vi "DB Set Measurement.vi"(4 "KH serial number":string, 5 "measurement":string, 6 "lockin serial number":string, 7 "device":string, 8 "error in (no error)":errorcluster, 9 "Station":string, 10 "User":string) -> (0 "error out":errorcluster)   [LabVIEW 2019, in "Control Experiment.lvclass"]
uses:
  Control Experiment.lvclass
  <userlib>/LevyLab/LV-Data/LV-Data.PG/LV-Data.PGSQL.lvclass
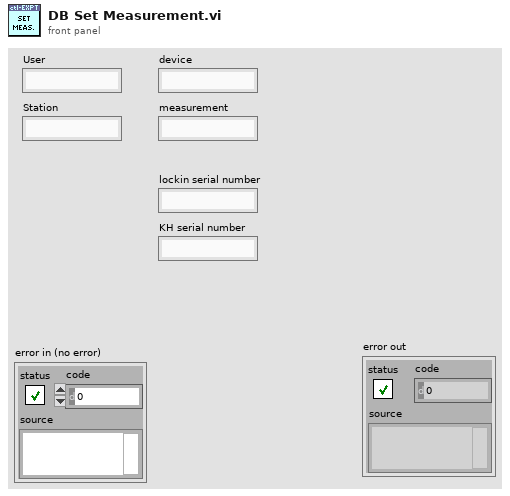
[diagram p1: front panel]
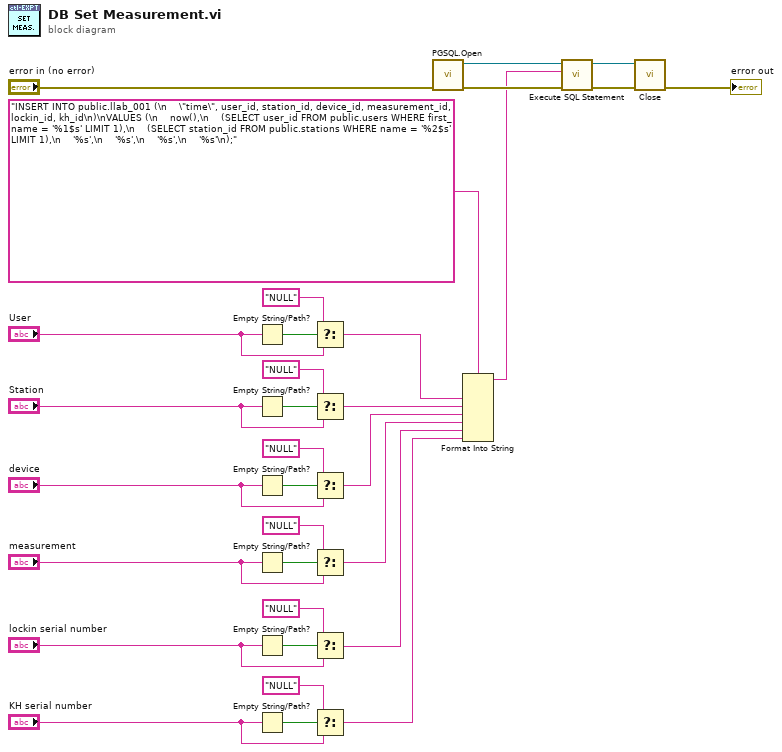
[diagram p0: block diagram]
diagram:
  n1 = Empty String/Path?(string/path="User") -> (empty?=w26:bool)
  n2 = Empty String/Path?(string/path="Station") -> (empty?=w31:bool)
  n3 = Empty String/Path?(string/path="device") -> (empty?=w15:bool)
  n4 = Empty String/Path?(string/path="measurement") -> (empty?=w12:bool)
  n5 = Empty String/Path?(string/path="lockin serial number") -> (empty?=w4:bool)
  n6 = Empty String/Path?(string/path="KH serial number") -> (empty?=w6:bool)
  n7 = Select(t="NULL", s=w26, f="User") -> (s? t:f=w24:string)
  n8 = Select(t="NULL", s=w31, f="Station") -> (s? t:f=w30:string)
  n9 = Select(t="NULL", s=w15, f="device") -> (s? t:f=w13:string)
  n10 = Select(t="NULL", s=w12, f="measurement") -> (s? t:f=w9:string)
  n11 = Select(t="NULL", s=w4, f="lockin serial number") -> (s? t:f=w2:string)
  n12 = Select(t="NULL", s=w6, f="KH serial number") -> (s? t:f=w1:string)
  n13 = call <userlib>:"PGSQL.Open.vi"("error in (no error)"="error in (no error)") -> ("error out"=w22:errorcluster, "Data.PG out"=w23:refnum<class "LV-Data.PGSQL.lvclass">)  [unwired: 9 in]
  n14 = Format Into String(format string="INSERT INTO public.llab_001 (\n    \"time\", user_id, station_id, device_id, measurement_id, lockin_id, kh_id\n)\nVALUES (\n    now(),\n    (SELECT user_id FROM public.users WHERE first_name = '%1$s' LIMIT 1),\n    (SELECT station_id FROM public.stations WHERE name = '%2$s' LIMIT 1),\n    '%s',\n    '%s',\n    '%s',\n    '%s'\n);" ("Address"), w24, w30, w13, w9, w2, w1) -> (resulting string=w21:string)  [unwired: 2 in, 1 out]
  n15 = call <userlib>:"Execute SQL Statement.vi"("error in (no error)"=w22, "SQL string"=w21, "Data.PGQL in"=w23) -> ("error out"=w20:errorcluster, "Data.PGSQL out"=w19:refnum<class "LV-Data.PGSQL.lvclass">)  [unwired: 6 in, 1 out]
  n16 = call-dynamic "Close.vi"("error in (no error)"=w20, "Data.PG in"=w19) -> ("error out"=→"error out":errorcluster)  [unwired: 8 in, 1 out]
